vi "Smooth derivative filter.vi"(7 "dt":dbl=0.05 format="%#_13g", 8 "Error In":errorcluster, 11 "Strain data":dbl[](array[numeric])=[0.0, 0.0, 0.0, 0.0, 0.0, 0.0, 0.0, 0.0, 0.0, 0.0, 0.0, 0.0]) -> (0 "Error Out":errorcluster, 3 "dStrain/dt":dbl[](array[numeric]))   [LabVIEW 2016]
uses:
  <vilib>/ptbypt/NI_PtbyPt.lvlib
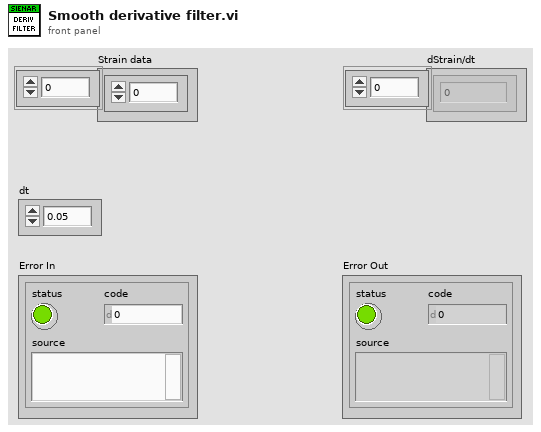
[diagram p1: front panel]
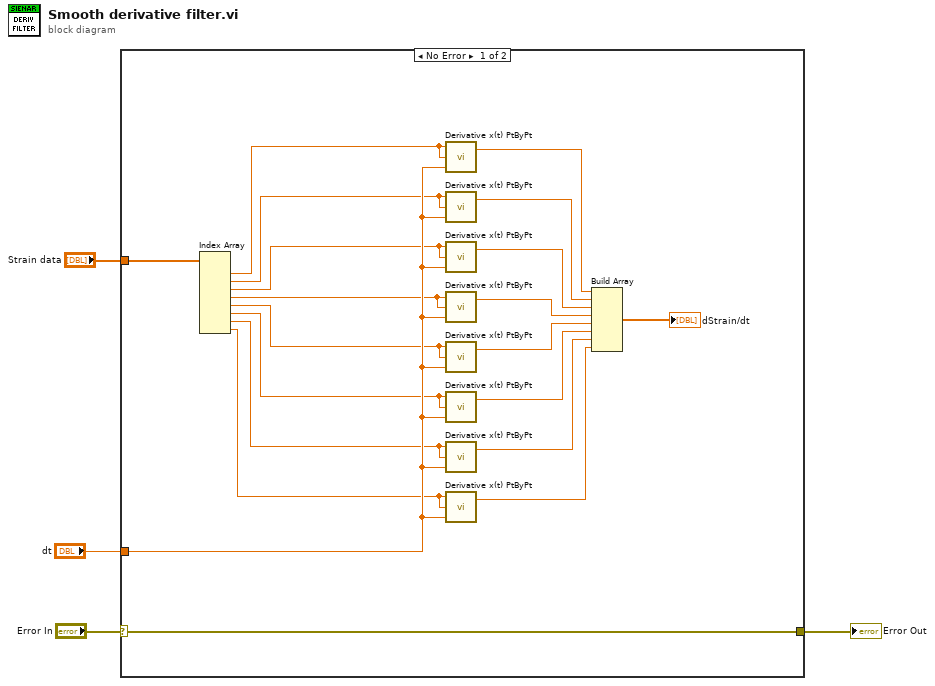
[diagram p0: block diagram]
diagram:
  n1 = case shown="No Error" "Error In" {
    selector: "Error In" -> [w24 w25]
    tunnel: "dt" -> [w22 _]
    tunnel: [w24 w25] -> w2
    tunnel: "Strain data" -> [w23 _]
    frame No Error {
      n2 = Index Array(array=w23) -> (element #1=w21:dbl, element #2=w20:dbl, element #3=w19:dbl, element #4=w18:dbl, element #5=w17:dbl, element #6=w16:dbl, element #7=w15:dbl, element #8=w14:dbl)  [unwired: 8 in]
      n3 = call <vilib>:"Derivative x(t) PtByPt.vi"("dt"=w22, "initial condition"=w21, "x"=w21) -> ("dx/dt"=w13:dbl)  [unwired: 1 in, 1 out]
      n4 = call <vilib>:"Derivative x(t) PtByPt.vi"("dt"=w22, "initial condition"=w20, "x"=w20) -> ("dx/dt"=w12:dbl)  [unwired: 1 in, 1 out]
      n5 = call <vilib>:"Derivative x(t) PtByPt.vi"("dt"=w22, "initial condition"=w19, "x"=w19) -> ("dx/dt"=w11:dbl)  [unwired: 1 in, 1 out]
      n6 = call <vilib>:"Derivative x(t) PtByPt.vi"("dt"=w22, "initial condition"=w18, "x"=w18) -> ("dx/dt"=w10:dbl)  [unwired: 1 in, 1 out]
      n7 = call <vilib>:"Derivative x(t) PtByPt.vi"("dt"=w22, "initial condition"=w17, "x"=w17) -> ("dx/dt"=w9:dbl)  [unwired: 1 in, 1 out]
      n8 = call <vilib>:"Derivative x(t) PtByPt.vi"("dt"=w22, "initial condition"=w16, "x"=w16) -> ("dx/dt"=w8:dbl)  [unwired: 1 in, 1 out]
      n9 = call <vilib>:"Derivative x(t) PtByPt.vi"("dt"=w22, "initial condition"=w15, "x"=w15) -> ("dx/dt"=w7:dbl)  [unwired: 1 in, 1 out]
      n10 = call <vilib>:"Derivative x(t) PtByPt.vi"("dt"=w22, "initial condition"=w14, "x"=w14) -> ("dx/dt"=w6:dbl)  [unwired: 1 in, 1 out]
      n11 = Build Array(w13, w12, w11, w10, w9, w8, w7, w6) -> (→"dStrain/dt":dbl[])
    }
    frame Error {
    }
  }
  "Error Out" <- w2
